vi "初始化.vi"(8 "error in (no error)":errorcluster caption="错误输入（无错误）", 9 "数据":T1, 11 "程序 输入":refnum<class "程序.lvclass">) -> (0 "error out":errorcluster caption="错误输出", 3 "程序 输出":refnum<class "程序.lvclass">)   [LabVIEW 2020, in "程序.lvclass"]
uses:
  D:/SuperPython-master/AutocompleteMenu-ScintillaNET.dll
  AutocompleteMenu-ScintillaNET.dll
  D:/SuperPython-master/ScintillaNET.dll
  ScintillaNET.dll
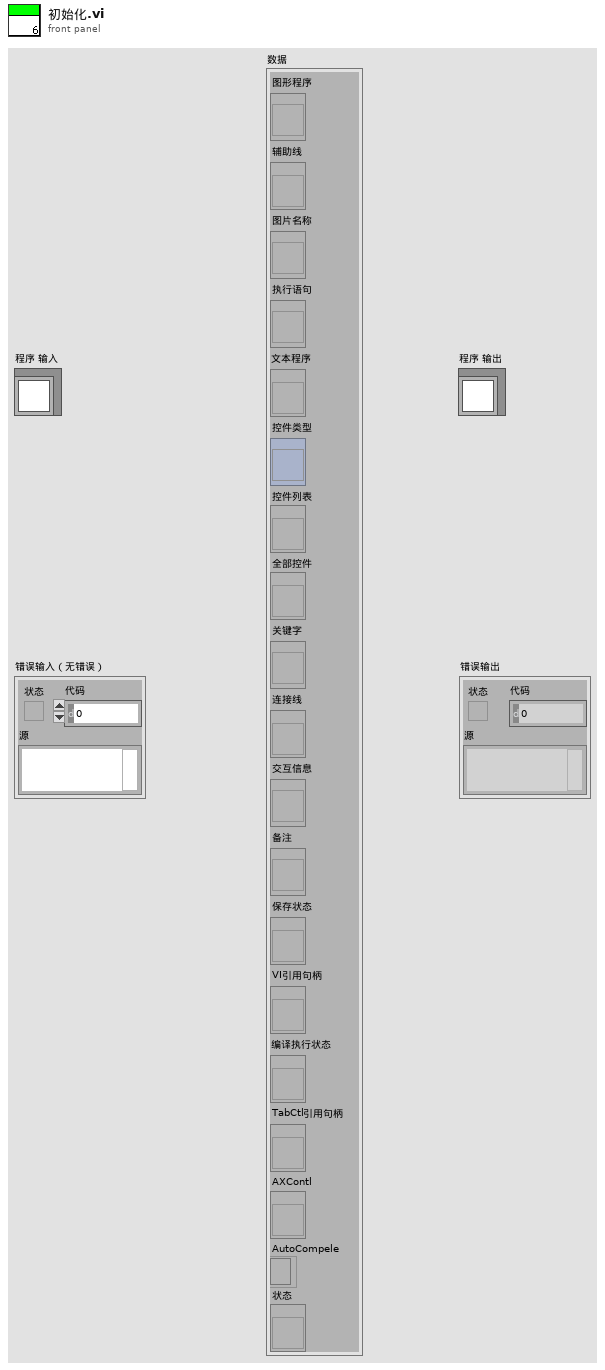
[diagram p1: front panel]
types:
  T1 = cluster{"图形程序":refnum<vi>, "辅助线":refnum<vi>, "图片名称":refnum<vi>, "执行语句":refnum<vi>, "文本程序":refnum<vi>, "控件类型":refnum<vi>, "控件列表":refnum<vi>, "全部控件":refnum<vi>, "关键字":refnum<vi>, "连接线":refnum<vi>, "交互信息":refnum<vi>, "备注":refnum<vi>, "保存状态":refnum<vi>, "VI引用句柄":refnum<vi>, "编译执行状态":refnum<vi>, "TabCtl引用句柄":refnum<vi>, "AXContl":refnum<vi>, "AutoCompele":refnum<k24>, "状态":refnum<vi>}
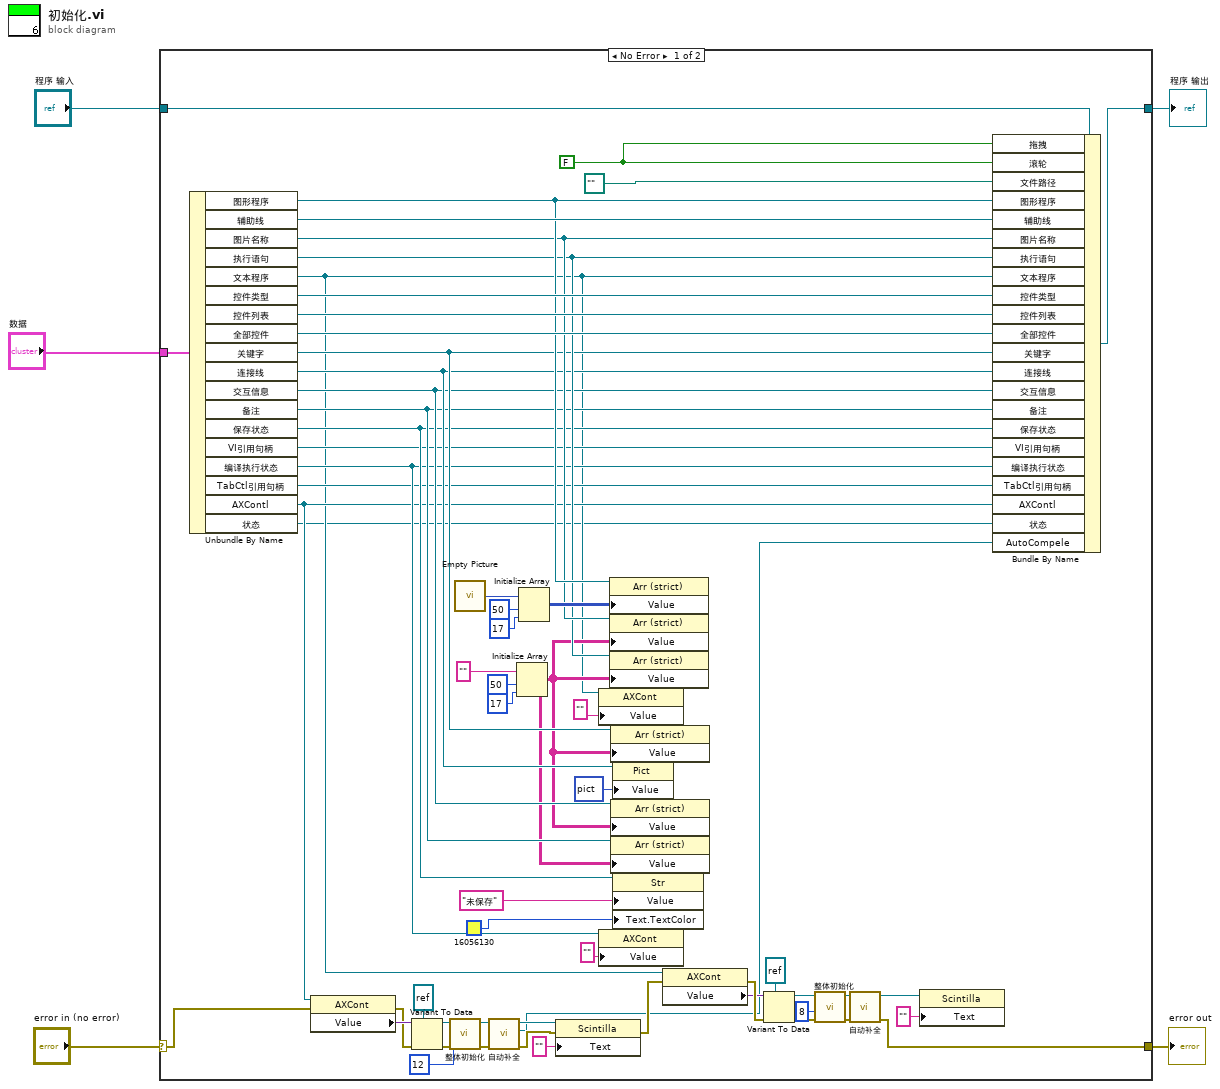
[diagram p0: block diagram]
diagram:
  n1 = case shown="No Error" "error in (no error)" {
    selector: "error in (no error)" -> [w17 w68]
    tunnel: [w16 w68] -> w4
    tunnel: [w65 w67] -> w2
    tunnel: "程序 输入" -> [w66 w67]
    tunnel: "数据" -> [w64 _]
    frame No Error {
      w37 = FALSE ("滚轮")
      n2 = Unbundle By Name(w64) -> ("图形程序"=w59:refnum<vi>, "辅助线"=w63:refnum<vi>, "图片名称"=w53:refnum<vi>, "执行语句"=w50:refnum<vi>, "文本程序"=w18:refnum<vi>, "控件类型"=w62:refnum<vi>, "控件列表"=w61:refnum<vi>, "全部控件"=w60:refnum<vi>, "关键字"=w48:refnum<vi>, "连接线"=w47:refnum<vi>, "交互信息"=w45:refnum<vi>, "备注"=w44:refnum<vi>, "保存状态"=w41:refnum<vi>, "VI引用句柄"=w38:refnum<vi>, "编译执行状态"=w35:refnum<vi>, "TabCtl引用句柄"=w32:refnum<vi>, "AXContl"=w31:refnum<vi>, "状态"=w15:refnum<vi>)
      n3 = property class="AXCont"(reference=w31, error in=w17) -> (error out=w26:errorcluster, "Value"=w30:variant)  [unwired: 1 out]
      n4 = Variant To Data(error in=w26, type=refnum<k24> refnum ("Scintilla"), Variant=w30) -> (data=w28:refnum<k24>, error out=w27:errorcluster)
      n5 = call "整体初始化.vi"("错误输入（无错误）"=w27, "大小"=12, "Scintilla"=w28) -> ("错误输出"=w33:errorcluster, "引用输出"=w34:refnum<k24>)  [unwired: 7 in]
      n6 = call "Empty Picture"() -> ("empty picture"=w56:picture)
      n7 = call "自动补全.vi"("错误输入"=w33, "引用"=w34) -> ("错误输出"=w10:errorcluster, "引用输出 2"=w8:refnum<k24>, "引用输出"=w14:refnum<k24>)  [unwired: 7 in]
      n8 = Initialize Array("", 50 ("维数大小"), 17 ("维数大小")) -> (w43:string[][])
      n9 = Initialize Array(w56, 50 ("维数大小"), 17 ("维数大小")) -> (w55:picture[][])
      n10 = property class="Scintilla"(reference=w14, error in=w10, "Text"="") -> (error out=w9:errorcluster)  [unwired: 1 out]
      n11 = property class="AXCont"(reference=w18, "Value"="" ("值")) -> ()  [unwired: 1 in, 2 out]
      n12 = property class="AXCont"(reference=w35, "Value"="" ("值")) -> ()  [unwired: 1 in, 2 out]
      n13 = property class="Arr (strict)"(reference=w59, "Value"=w55) -> ()  [unwired: 1 in, 2 out]
      n14 = property class="Arr (strict)"(reference=w53, "Value"=w43) -> ()  [unwired: 1 in, 2 out]
      n15 = property class="Arr (strict)"(reference=w50, "Value"=w43) -> ()  [unwired: 1 in, 2 out]
      n16 = property class="Arr (strict)"(reference=w48, "Value"=w43) -> ()  [unwired: 1 in, 2 out]
      n17 = property class="Arr (strict)"(reference=w45, "Value"=w43) -> ()  [unwired: 1 in, 2 out]
      n18 = property class="Arr (strict)"(reference=w44, "Value"=w43) -> ()  [unwired: 1 in, 2 out]
      n19 = property class="Pict"(reference=w47, "Value"=picture data[5B] ("值")) -> ()  [unwired: 1 in, 2 out]
      n20 = property class="Str"(reference=w41, "Value"="未保存" ("值"), "Text.TextColor"=u32 16056130) -> ()  [unwired: 1 in, 2 out]
      n21 = property class="AXCont"(reference=w18, error in=w9) -> (error out=w25:errorcluster, "Value"=w21:variant)  [unwired: 1 out]
      n22 = Variant To Data(error in=w25, type=refnum<k24> refnum ("Scintilla"), Variant=w21) -> (data=w23:refnum<k24>, error out=w24:errorcluster)
      n23 = call "整体初始化.vi"("错误输入（无错误）"=w24, "大小"=8, "Scintilla"=w23) -> ("错误输出"=w20:errorcluster, "引用输出"=w19:refnum<k24>)  [unwired: 7 in]
      n24 = call "自动补全.vi"("错误输入"=w20, "引用"=w19) -> ("错误输出"=w16:errorcluster, "引用输出"=w12:refnum<k24>)  [unwired: 7 in, 1 out]
      n25 = property class="Scintilla"(reference=w12, "Text"="") -> ()  [unwired: 1 in, 2 out]
      n26 = Bundle By Name(cluster=w66, "拖拽"=w37, "滚轮"=w37, "文件路径"=path "", "图形程序"=w59, "辅助线"=w63, "图片名称"=w53, "执行语句"=w50, "文本程序"=w18, "控件类型"=w62, "控件列表"=w61, "全部控件"=w60, "关键字"=w48, "连接线"=w47, "交互信息"=w45, "备注"=w44, "保存状态"=w41, "VI引用句柄"=w38, "编译执行状态"=w35, "TabCtl引用句柄"=w32, "AXContl"=w31, "状态"=w15, "AutoCompele"=w8) -> (w65:refnum<class "程序.lvclass">)
    }
    frame Error {
    }
  }
  "error out" <- w4
  "程序 输出" <- w2
